vi "OnTick.vi"(8 "Uart Input":cluster{u64} {"?" format="%x"}, 11 "Error Input":errorcluster) -> (0 "Uart Output":cluster{u64} {"?" format="%x"}, 2 "On Tick Event":refnum<event-registration>, 3 "Error Output":errorcluster)   [LabVIEW 2019]
doc: "Add an <B>On Tick Received</B> event listener to the serial port."
uses:
  dll/LabViewUart.dll
panel:
  # "Add an On_Tick event listenner"
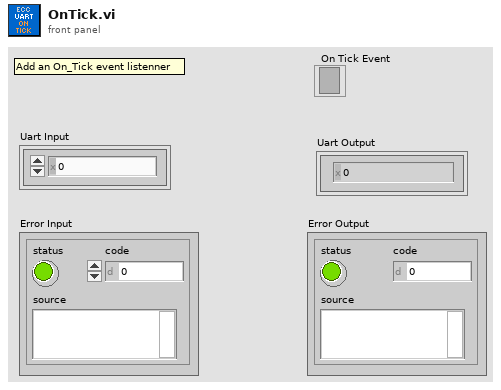
[diagram p1: front panel]
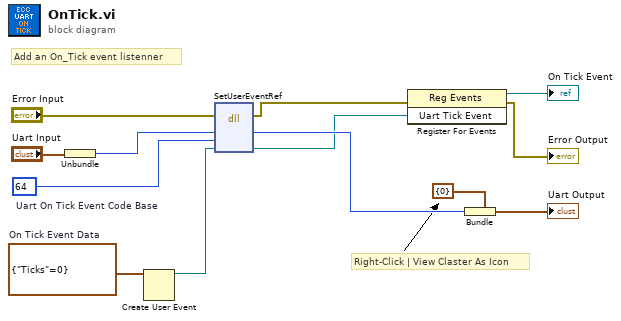
[diagram p0: block diagram]
diagram:
  w10 = cluster{"Ticks":u32} {"Ticks"=0}  # On Tick Event Data
  w13 = u16 64  # Uart On Tick Event Code Base
  # "Right-Click | View Claster As Icon"
  # "Add an On_Tick event listenner"
  n1 = Unbundle("Uart Input") -> (w5:u64)
  n2 = Create User Event(user event datatype=w10) -> (user event=w12:refnum<user-event>)  [unwired: 1 in, 1 out]
  n3 = dll-call lib="D:/Google Drive/INC-2020/INC352/INC352-2020/LabVIEW/examples/uart-cmdex/SubVI/dll/LabViewUart.dll" fn="SetUserEventRef"(error in="Error Input", "Uart Handle"=w5, "Uart On Tick Event Code Base"=w13, "Uart Tick Event"=w12) -> (error out=w2:errorcluster, "Uart Handle"=w8:u64, "Uart Tick Event"=w4:refnum<user-event>)  [unwired: 4 in, 1 out]
  n4 = register-events(error in=w2, w4) -> (reference out=→"On Tick Event":refnum<event-registration>, error out=→"Error Output":errorcluster)  [unwired: 1 in]
  n5 = Bundle(cluster=cluster{u64} {0}, w8) -> (→"Uart Output":cluster{u64})
